vi "Set fixed_coords.vi"(11 "eu data in":dbl[](array[numeric])) -> (1 "valid":bool=TRUE, 3 "raw data out":u8[](array[numeric]))   [LabVIEW 2019, in "HLA Data Conversion.lvlib"]
uses:
  HLA Data Conversion.lvlib
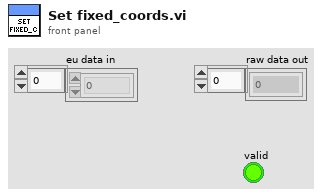
[diagram p1: front panel]
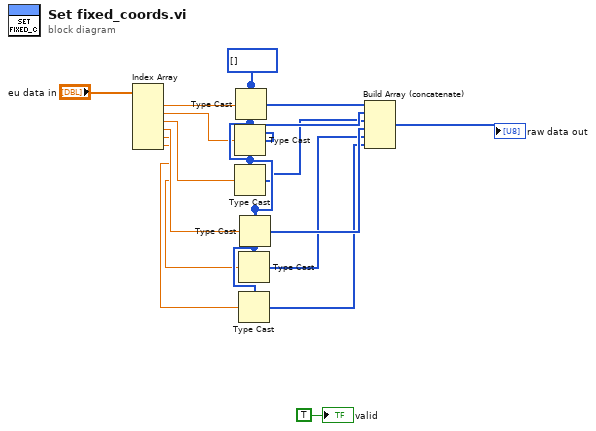
[diagram p0: block diagram]
diagram:
  w11 = u8[] [] ("raw data out")
  n1 = Index Array(array="eu data in") -> (element #1=w14:dbl, element #2=w10:dbl, element #3=w9:dbl, element #4=w8:dbl, element #5=w7:dbl, element #6=w6:dbl)  [unwired: 6 in]
  n2 = Type Cast(type=w11, x=w10) -> (*(type *) &x=w5:u8[])
  n3 = Type Cast(type=w11, x=w9) -> (*(type *) &x=w4:u8[])
  n4 = Type Cast(type=w11, x=w14) -> (*(type *) &x=w13:u8[])
  n5 = Type Cast(type=w11, x=w7) -> (*(type *) &x=w2:u8[])
  n6 = Type Cast(type=w11, x=w6) -> (*(type *) &x=w1:u8[])
  n7 = Type Cast(type=w11, x=w8) -> (*(type *) &x=w3:u8[])
  n8 = Build Array (concatenate)(w13, w5, w4, w3, w2, w1) -> (→"raw data out":u8[])
  "valid" <- TRUE
